vi "Configure DC Volts5.vi"(8 "error in (no error)":errorcluster, 10 "measurementservice_DMMConfigRequest_Data":T3, 11 "DMMSession":refnum<k15>) -> (0 "error out":errorcluster, 2 "measurementservice_DMMConfigResponse_Data":T1)   [LabVIEW 2019, in "HVC5.lvlib" / "HVC5.lvclass"]
uses:
  HVC5 Class/HVC5.lvclass
  <instrlib>/niDMM/nidmm.llb/niDMM Control Actions.ctl
  HVC5 Class/RPC Messages/measurementservice_ErrorOut/measurementservice_ErrorOut_Data.ctl
  HVC5 Class/RPC Messages/measurementservice_DMMConfigResponse/measurementservice_DMMConfigResponse_Data.ctl
  <instrlib>/niDMM/nidmm.llb/niDMM Configure Measurement Digits.vi
  HVC5 Class/RPC Messages/measurementservice_DMMConfigRequest/measurementservice_DMMConfigRequest_Data.ctl
panel:
  in  "DMM Function Array":i32[](array[numeric])=[1, 2, 3, 4, 5, 101, 1002, 104, 105, 1001, 1005, 1006, 108]
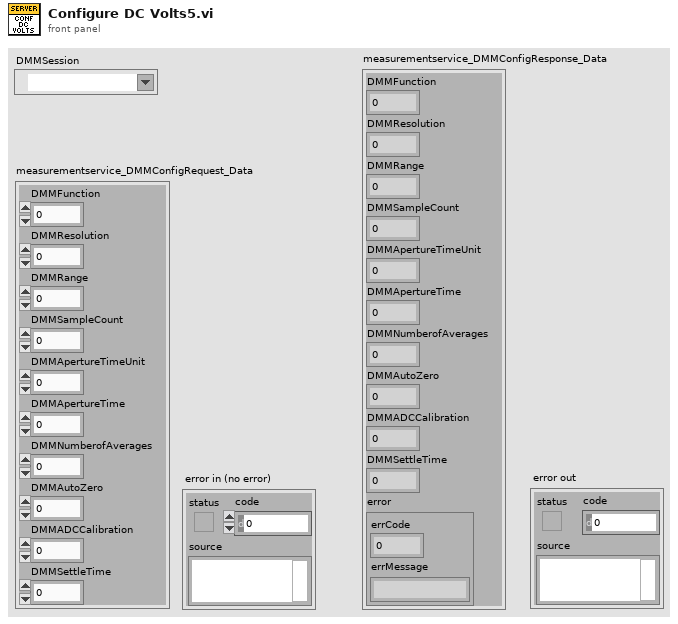
[diagram p1: front panel]
types:
  T1 = typedef "HVC5.lvlib/HVC5.lvclass/measurementservice_DMMConfigResponse_Data.ctl" = cluster{"DMMFunction":i32, "DMMResolution":sgl, "DMMRange":sgl, "DMMSampleCount":i32, "DMMApertureTimeUnit":i32, "DMMApertureTime":sgl, "DMMNumberofAverages":i32, "DMMAutoZero":i32, "DMMADCCalibration":i32, "DMMSettleTime":sgl, "error":T2}
  T2 = typedef "HVC5.lvlib/HVC5.lvclass/measurementservice_ErrorOut_Data.ctl" = cluster{"errCode":i32, "errMessage":string}
  T3 = typedef "HVC5.lvlib/HVC5.lvclass/measurementservice_DMMConfigRequest_Data.ctl" = cluster{"DMMFunction":i32, "DMMResolution":sgl, "DMMRange":sgl, "DMMSampleCount":i32, "DMMApertureTimeUnit":i32, "DMMApertureTime":sgl, "DMMNumberofAverages":i32, "DMMAutoZero":i32, "DMMADCCalibration":i32, "DMMSettleTime":sgl}
  T4 = typedef "niDMM Control Actions.ctl" = i32
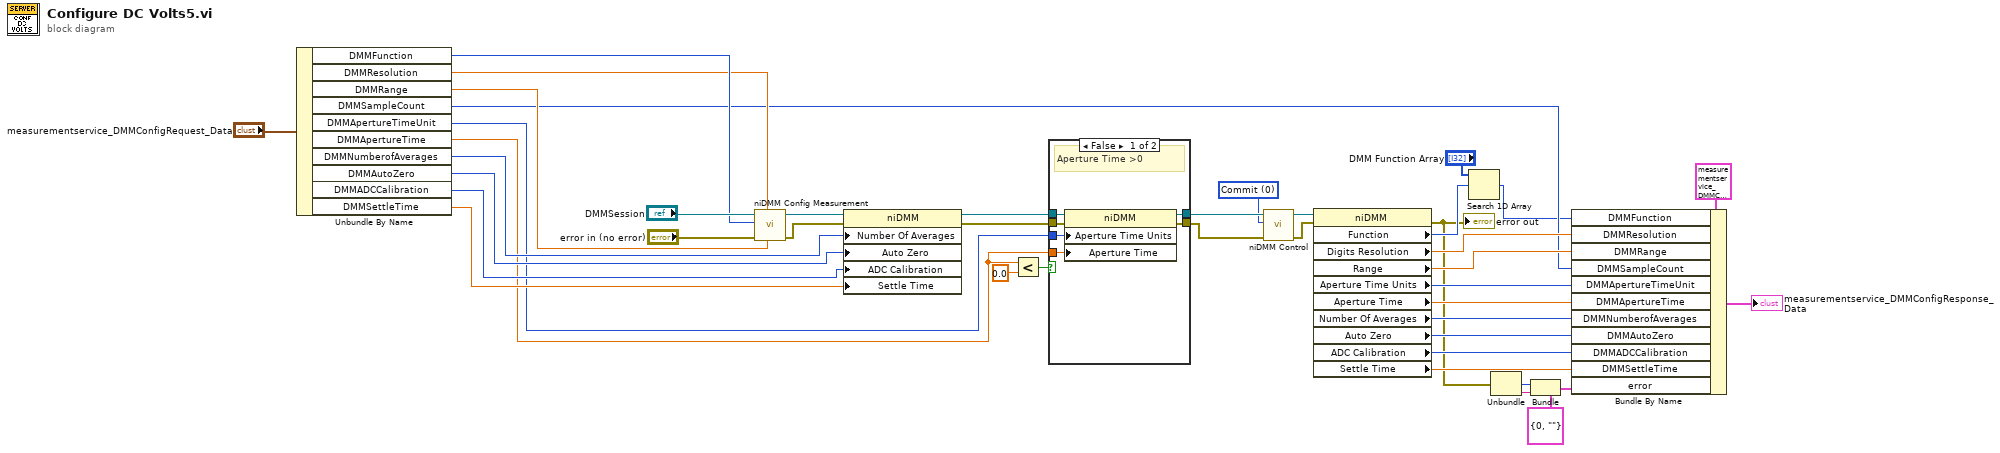
[diagram p0: block diagram]
diagram:
  w24 = T4 0 items=["Commit"] ("Control Action")
  n1 = Unbundle By Name("measurementservice_DMMConfigRequest_Data") -> ("DMMFunction"=w41:i32, "DMMResolution"=w40:sgl, "DMMRange"=w39:sgl, "DMMSampleCount"=w13:i32, "DMMApertureTimeUnit"=w28:i32, "DMMApertureTime"=w27:sgl, "DMMNumberofAverages"=w36:i32, "DMMAutoZero"=w35:i32, "DMMADCCalibration"=w34:i32, "DMMSettleTime"=w33:sgl)
  n2 = call-poly <instrlib>:"niDMM Config Measurement.vi"("Range"=w39, "Resolution in Digits"=w40, "error in (no error)"="error in (no error)", "Function"=w41, "instrument handle"="DMMSession") -> ("error out"=w37:errorcluster, "instrument handle out"=w38:refnum<k15>)  [unwired: 5 in]
  n3 = property class="niDMM"(reference=w38, error in=w37, "Number Of Averages"=w36, "Auto Zero"=w35, "ADC Calibration"=w34, "Settle Time"=w33) -> (reference out=w32:refnum<k15>, error out=w31:errorcluster)
  n4 = Less?(x=w27, y=0.0 ("Configuration:Advanced:Aperture Time")) -> (x < y?=w29:bool)
  n5 = case shown="False" w29 {
    tunnel: w32 -> [w48 w50]
    tunnel: w31 -> [w47 w49]
    tunnel: [w46 w50] -> w26
    tunnel: [w45 w49] -> w25
    tunnel: w28 -> [w44 _]
    tunnel: w27 -> [w43 _]
    frame False {
      # "Aperture Time >0"
      n6 = property class="niDMM"(reference=w48, error in=w47, "Aperture Time Units"=w44, "Aperture Time"=w43) -> (reference out=w46:refnum<k15>, error out=w45:errorcluster)
    }
    frame True {
      # "Aperture Time <0"
    }
  }
  n7 = call <instrlib>:"niDMM Control.vi"("error in (no error)"=w25, "Control Action"=w24, "instrument handle"=w26) -> ("error out"=w22:errorcluster, "instrument handle out"=w23:refnum<k15>)  [unwired: 7 in]
  n8 = property class="niDMM"(reference=w23, error in=w22) -> (error out=w1:errorcluster, "Function"=w11:i32, "Digits Resolution"=w14:dbl, "Range"=w15:dbl, "Aperture Time Units"=w16:i32, "Aperture Time"=w17:dbl, "Number Of Averages"=w18:i32, "Auto Zero"=w19:i32, "ADC Calibration"=w20:i32, "Settle Time"=w21:dbl)  [unwired: 1 out]
  "error out" <- w1
  n9 = Search 1D Array(1D array="DMM Function Array", element=w11) -> (index of element=w10:i32)  [unwired: 1 in]
  n10 = Unbundle(w1) -> ("code"=w4:i32, "source"=w3:string)  [unwired: 1 out]
  n11 = Bundle(cluster=T2 {"errCode"=0, "errMessage"=""} ("error"), "errCode"=w4, "errMessage"=w3) -> (w5:T2)
  n12 = Bundle By Name(cluster=T1 {"DMMFunction"=0, "DMMResolution"=0.0, "DMMRange"=0.0, "DMMSampleCount"=0, "DMMApertureTimeUnit"=0, "DMMApertureTime"=0.0, "DMMNumberofAverages"=0, "DMMAutoZero"=0, "DMMADCCalibration"=0, "DMMSettleTime"=0.0, "error"={"errCode"=0, "errMessage"=""}} ("measurementservice_DMMConfigResponse_Data"), "DMMFunction"=w10, "DMMResolution"=w14, "DMMRange"=w15, "DMMSampleCount"=w13, "DMMApertureTimeUnit"=w16, "DMMApertureTime"=w17, "DMMNumberofAverages"=w18, "DMMAutoZero"=w19, "DMMADCCalibration"=w20, "DMMSettleTime"=w21, "error"=w5) -> (→"measurementservice_DMMConfigResponse_Data":T1)
